vi "conv_with_kernel.vi"(10 "Kernel":dbl[][](array[numeric])=[[0.1111111, 0.1111111, 0.1111111], [0.1111111, 0.1111111, 0.1111111], [0.1111111, 0.1111111, 0.1111111]], 11 "Image":T1) -> (3 "Proccessed image":T1)   [LabVIEW 2022 SP3]
doc: "Perfoms convolution on image with given kernel (2D array). Returns image after convolution."
uses:
  <vilib>/picture/picture.llb/imagedata.ctl
  <vilib>/Analysis/2dsp.llb/2D Convolution (DBL).vi
  <vilib>/picture/picture.llb/Draw True-Color Pixmap.vi
  <vilib>/Analysis/NI_AALPro.lvlib
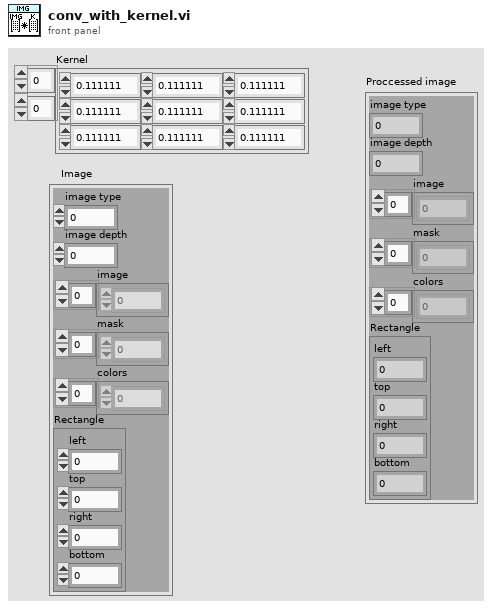
[diagram p1: front panel]
types:
  T1 = typedef "imagedata.ctl" = cluster{"image type":i32, "image depth":i32, "image":u8[], "mask":u8[], "colors":u32[], "Rectangle":cluster{"left":i16, "top":i16, "right":i16, "bottom":i16}}
  T2 = cluster{"left":i16, "top":i16, "right":i16, "bottom":i16}
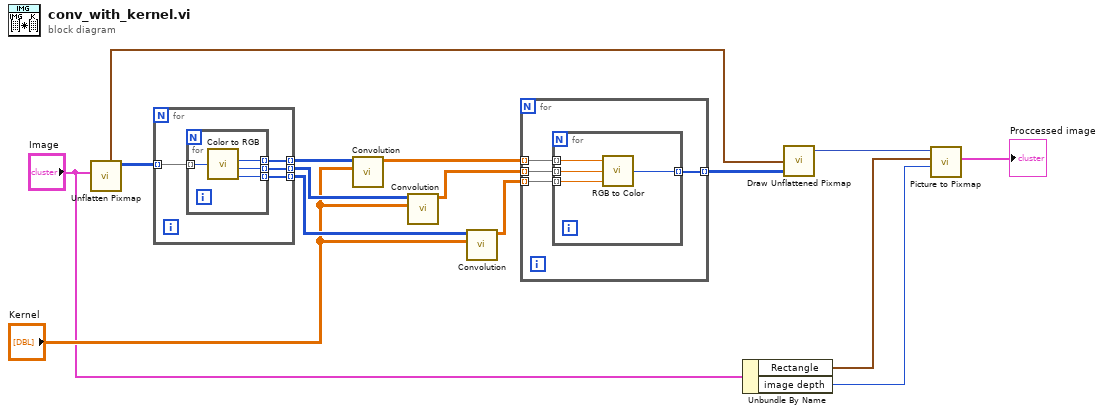
[diagram p0: block diagram]
diagram:
  n1 = call <vilib>:"Unflatten Pixmap.vi"("image data"="Image") -> ("24-bit pixmap"=w7:u32[][], "top left"=w8:cluster{"x":i16, "y":i16})  [unwired: 4 in, 5 out]
  n2 = for {
    tunnel: w7 -> [w19] mode=indexing
    tunnel: [w18] -> w15 mode=indexing
    tunnel: [w17] -> w14 mode=indexing
    tunnel: [w16] -> w13 mode=indexing
    n3 = for {
      tunnel: w19 -> [w23] mode=indexing
      tunnel: [w22] -> w18 mode=indexing
      tunnel: [w21] -> w17 mode=indexing
      tunnel: [w20] -> w16 mode=indexing
      n4 = call <vilib>:"Color to RGB.vi"("Color"=w23) -> ("R"=w22:u8, "G"=w21:u8, "B"=w20:u8)  [unwired: 1 out]
    }
  }
  n5 = call-poly <vilib>:"Convolution.vi"("Y"="Kernel", "X"=w15) -> ("X * Y"=w11:dbl[][])  [unwired: 8 in, 1 out]
  n6 = call-poly <vilib>:"Convolution.vi"("Y"="Kernel", "X"=w14) -> ("X * Y"=w10:dbl[][])  [unwired: 8 in, 1 out]
  n7 = call-poly <vilib>:"Convolution.vi"("Y"="Kernel", "X"=w13) -> ("X * Y"=w9:dbl[][])  [unwired: 8 in, 1 out]
  n8 = for {
    tunnel: w11 -> [w27] mode=indexing
    tunnel: w10 -> [w26] mode=indexing
    tunnel: w9 -> [w25] mode=indexing
    tunnel: [w24] -> w1 mode=indexing
    n9 = for {
      tunnel: w27 -> [w31] mode=indexing
      tunnel: w26 -> [w30] mode=indexing
      tunnel: w25 -> [w29] mode=indexing
      tunnel: [w28] -> w24 mode=indexing
      n10 = call <vilib>:"RGB to Color.vi"("B"=w29, "G"=w30, "R"=w31) -> ("Color"=w28:u32)
    }
  }
  n11 = Unbundle By Name("Image") -> ("Rectangle"=w4:T2, "image depth"=w3:i32)
  n12 = call-poly <vilib>:"Draw Unflattened Pixmap.vi"("top left point(0, 0)"=w8, "data (RGB format)"=w1) -> ("new picture"=w6:picture)  [unwired: 7 in]
  n13 = call <vilib>:"Picture to Pixmap.vi"("depth"=w3, "rect"=w4, "picture"=w6) -> ("image data"=→"Proccessed image":T1)  [unwired: 7 in, 1 out]
